vi "parse_vehicle_status.vi"(8 "error in":errorcluster, 11 "msg in":string) -> (0 "error out":errorcluster, 2 "vehicle_status":T1, 3 "msg out":string)   [LabVIEW 2016]
uses:
  <userlib>/ROS for LabVIEW Software/ROS/MessageParsing/std_msgs/subs/parse_float64_scalar.vi
  <userlib>/ROS for LabVIEW Software/ROS/MessageParsing/std_msgs/subs/parse_i8_scalar.vi
  <userlib>/ROS for LabVIEW Software/ROS/MessageParsing/std_msgs/subs/parse_string_scalar.vi
  <userlib>/ROS for LabVIEW Software/ROS/MessageParsing/std_msgs/subs/parse_time_scalar.vi
  <userlib>/ROS for LabVIEW Software/ROS/MessageParsing/std_msgs/subs/parse_u64_scalar.vi
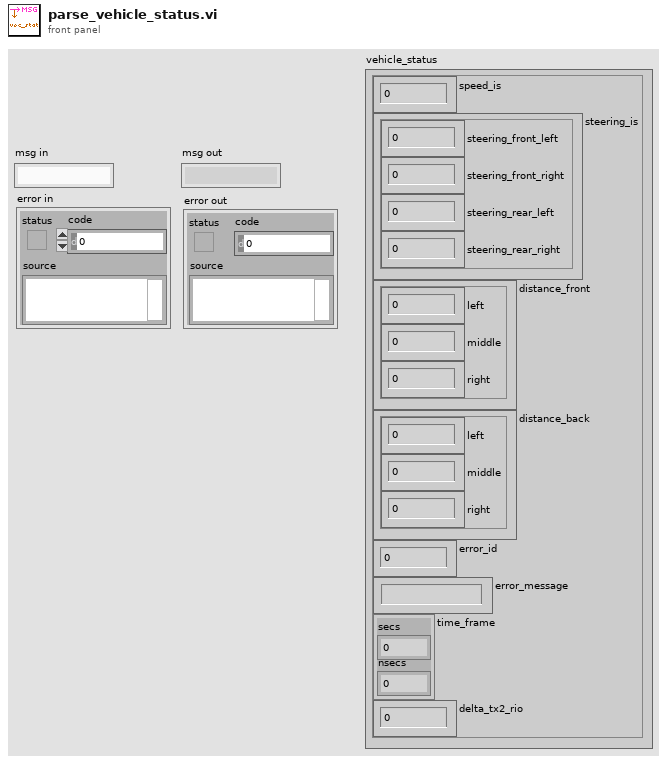
[diagram p1: front panel]
types:
  T1 = cluster{"speed_is":dbl, "steering_is":cluster{"steering_front_left":dbl, "steering_front_right":dbl, "steering_rear_left":dbl, "steering_rear_right":dbl}, "distance_front":cluster{"left":dbl, "middle":dbl, "right":dbl}, "distance_back":cluster{"left":dbl, "middle":dbl, "right":dbl}, "error_id":i8, "error_message":string, "time_frame":cluster{"secs":i32, "nsecs":i32}, "delta_tx2_rio":u64}
  T2 = cluster{"speed_is":dbl, "steering_is":cluster{"steering_front_left":dbl, "steering_front_right":dbl, "steering_rear_left":dbl, "steering_rear_right":dbl}, "distance_front":cluster{"Left":dbl, "Middle":dbl, "Right":dbl}, "distance_back":cluster{"Left":dbl, "Middle":dbl, "Right":dbl}, "error_id":i8, "error_message":string, "time_frame":cluster{"secs":i32, "nsecs":i32}, "delta_tx2_rio":u64}
  T3 = cluster{"steering_front_left":dbl, "steering_front_right":dbl, "steering_rear_left":dbl, "steering_rear_right":dbl}
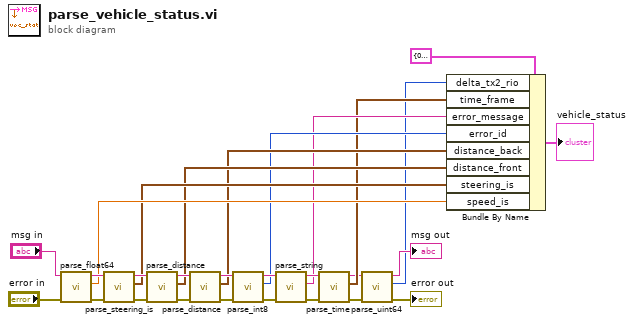
[diagram p0: block diagram]
diagram:
  n1 = call-poly <userlib>:"parse_float64.vi"("error in"="error in", "msg in"="msg in") -> ("error out"=w20:errorcluster, "number"=w13:dbl, "msg out"=w26:string)  [unwired: 3 in]
  n2 = call "parse_steering_is.vi"("error in"=w20, "msg in"=w26) -> ("error out"=w19:errorcluster, "steering_is"=w12:T3, "msg out"=w25:string)  [unwired: 7 in]
  n3 = call "parse_distance.vi"("error in"=w19, "msg in"=w25) -> ("error out"=w18:errorcluster, "distance"=w11:cluster{"Left":dbl, "Middle":dbl, "Right":dbl}, "msg out"=w24:string)  [unwired: 7 in]
  n4 = call "parse_distance.vi"("error in"=w18, "msg in"=w24) -> ("error out"=w17:errorcluster, "distance"=w10:cluster{"Left":dbl, "Middle":dbl, "Right":dbl}, "msg out"=w23:string)  [unwired: 7 in]
  n5 = call-poly <userlib>:"parse_int8.vi"("error in"=w17, "msg in"=w23) -> ("error out"=w16:errorcluster, "number"=w9:i8, "msg out"=w22:string)  [unwired: 3 in]
  n6 = call-poly <userlib>:"parse_string.vi"("error in"=w16, "msg in"=w22) -> ("error out"=w15:errorcluster, "string"=w8:string, "msg out"=w21:string)  [unwired: 3 in]
  n7 = call-poly <userlib>:"parse_time.vi"("error in"=w15, "msg in"=w21) -> ("error out"=w4:errorcluster, "Time"=w7:cluster{"secs":i32, "nsecs":i32}, "msg out"=w5:string)  [unwired: 3 in]
  n8 = call-poly <userlib>:"parse_uint64.vi"("error in"=w4, "msg in"=w5) -> ("error out"=→"error out":errorcluster, "number"=w1:u64, "msg out"=→"msg out":string)  [unwired: 3 in]
  n9 = Bundle By Name(cluster=T2 {"speed_is"=0.0, "steering_is"={"steering_front_left"=0.0, "steering_front_right"=0.0, "steering_rear_left"=0.0, "steering_rear_right"=0.0}, "distance_front"={"Left"=0.0, "Middle"=0.0, "Right"=0.0}, "distance_back"={"Left"=0.0, "Middle"=0.0, "Right"=0.0}, "error_id"=0, "error_message"="", "time_frame"={"secs"=0, "nsecs"=0}, "delta_tx2_rio"=0}, "delta_tx2_rio"=w1, "time_frame"=w7, "error_message"=w8, "error_id"=w9, "distance_back"=w10, "distance_front"=w11, "steering_is"=w12, "speed_is"=w13) -> (→"vehicle_status":T2)
